vi "BRig_dataExp_LED_baseline_l1.vi"() -> (2 "output_LED_baseline_l1":i32)   [LabVIEW 2014]
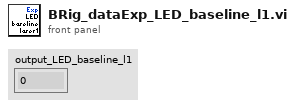
[diagram p1: front panel]
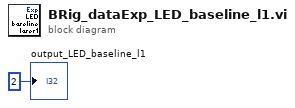
[diagram p0: block diagram]
diagram:
  "output_LED_baseline_l1" <- 2 ("output_iBlock")
